vi "KB-求内环平面点.vi"(10 "offset":i32, 11 "波形图 7":dbl[](array[numeric])=[0.0, 0.0, 3.9952999999999994, 3.9923, 3.9387999999999996, 3.8314999999999997, 3.7700000000000005, 3.7629000000000006, 3.7614999999999994, 3.7604999999999995, 3.7603999999999997, 3.7639000000000005, 3.7711999999999994, 0.0]) -> (2 "index":i32, 3 "元素":dbl)   [LabVIEW 2015]
panel:
  out "x/y":dbl
  out "已排序的数组 2":dbl[](array[numeric])
  out "已排序的数组":dbl[](array[numeric])
  out "最小值 2":dbl
  out "元素索引":i32
  out "最小索引 2":i32
  out "反转的数组 3":dbl[](array[numeric])
  out "反转的数组 2":dbl[](array[numeric])
  out "反转的数组":dbl[](array[numeric])
  out "最小索引":i32
  out "波形图 6":dbl[](graph)
  out "最小值":dbl
  out "波形图 5":dbl[](graph)
  out "数组":dbl[](array[numeric])
  out "波形图 4":dynamicdata(graph)
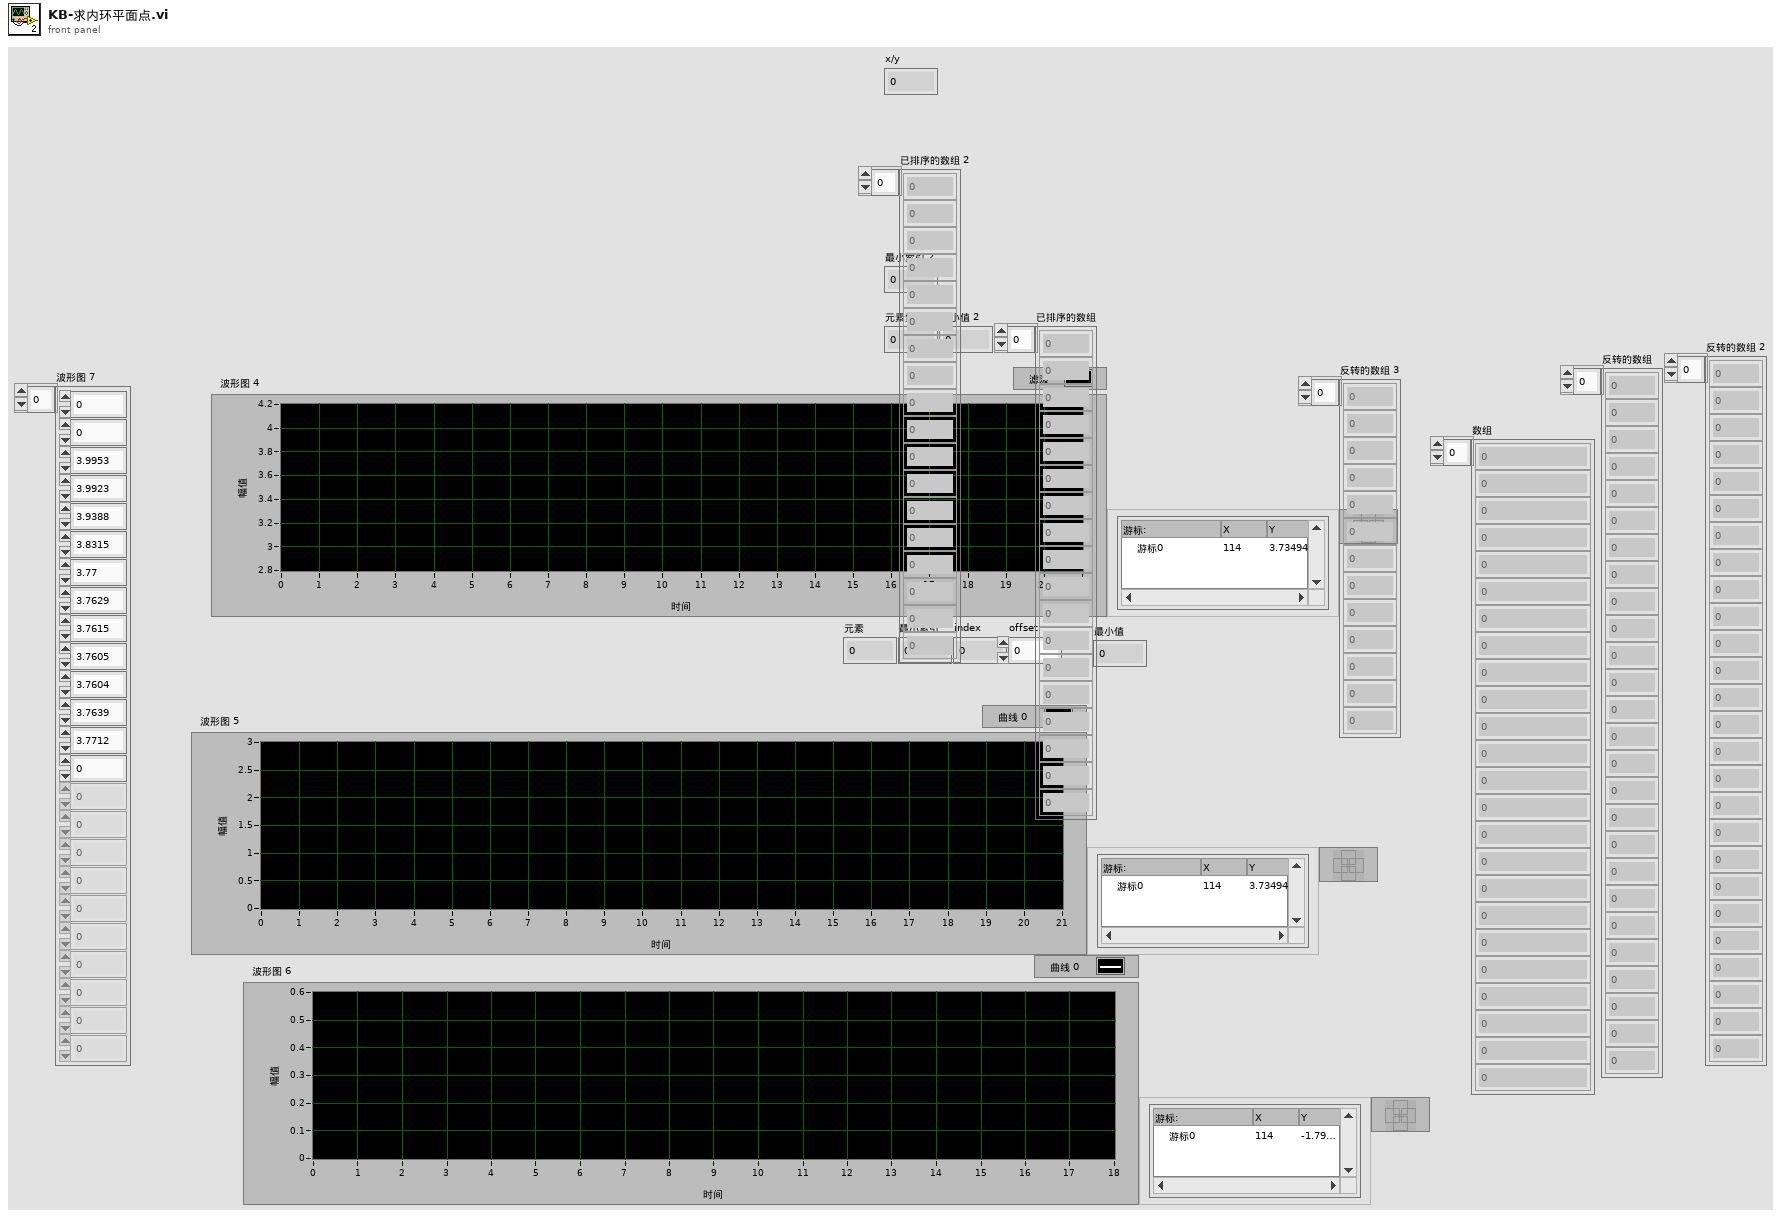
[diagram p1: front panel]
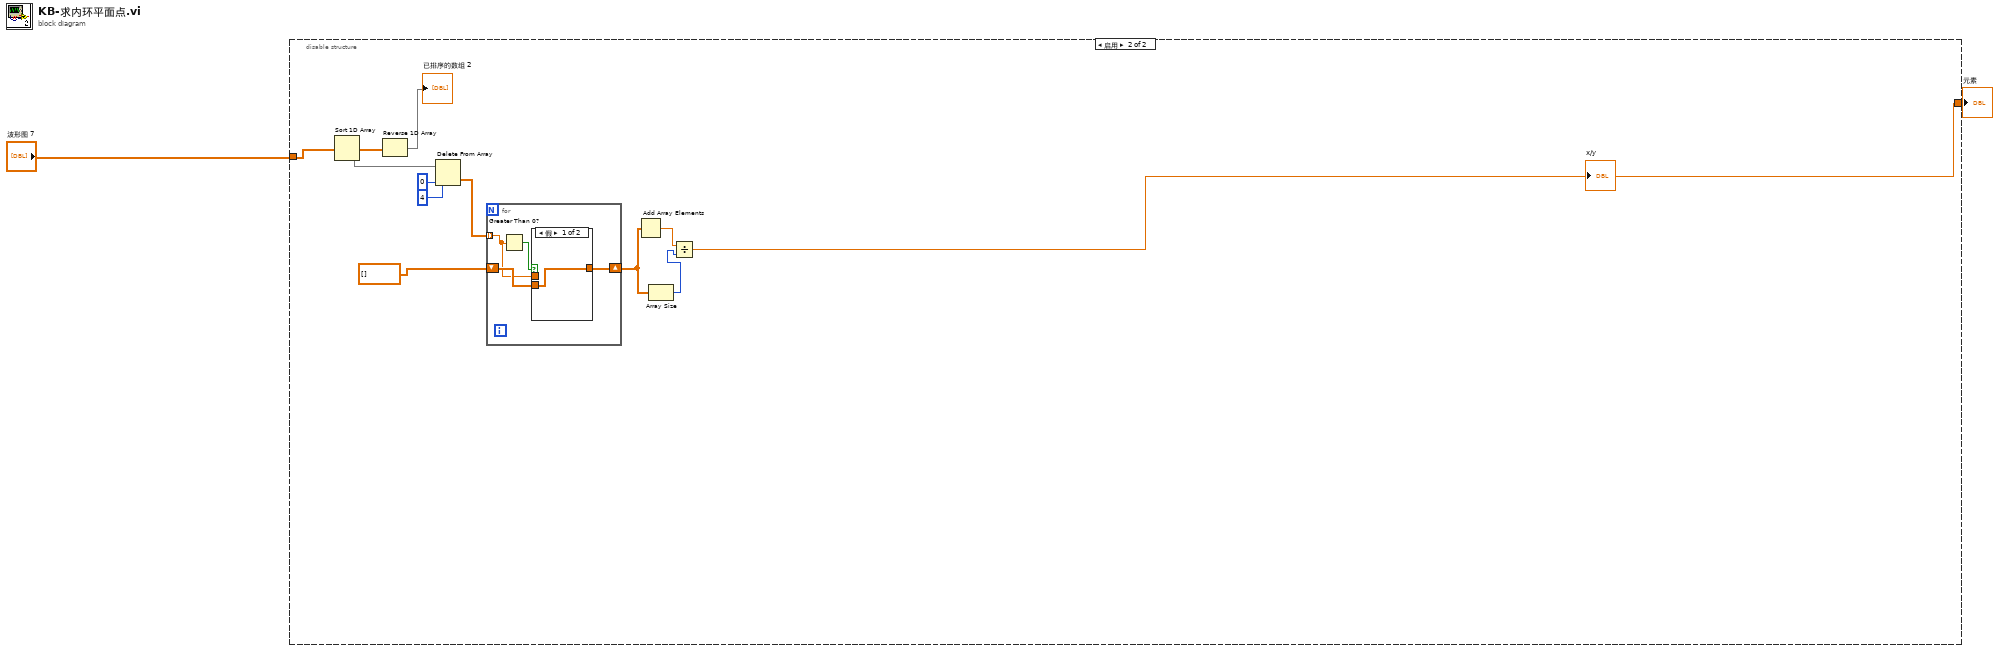
[diagram p0: block diagram]
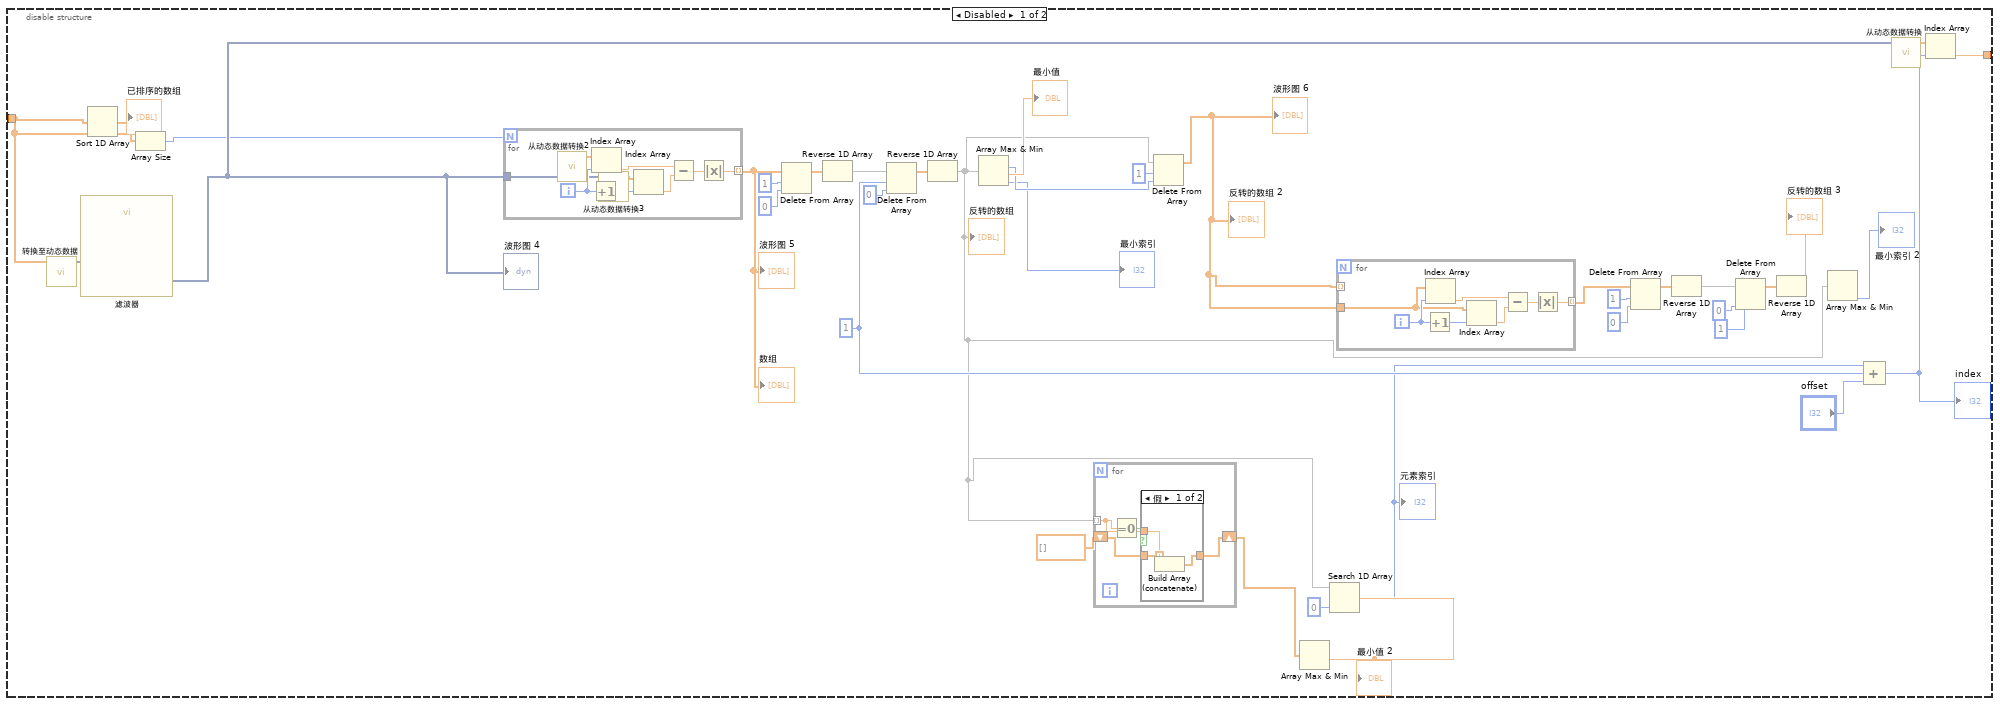
[diagram p2: hidden frame]
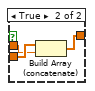
[diagram p4: hidden frame]
diagram:
  n1 = disable-structure shown="启用" {
    disable-tunnel: [w33 w69] -> w2
    disable-tunnel: "波形图 7" -> [w4 w75]
    frame Disabled {
      w32 = 1 ("长度")
      n2 = call "转换至动态数据"("Array"=w4) -> ("Dynamic Data Type"=w8:dynamicdata)  [unwired: 3 in]
      n3 = call "滤波器"("Signal"=w8) -> ("Filtered Signal"=w7:dynamicdata)  [unwired: 9 in, 1 out]
      "波形图 4" <- w7
      n4 = Sort 1D Array(array=w4) -> (sorted array=→"已排序的数组":dbl[])
      n5 = Array Size(array=w4) -> (size(s)=w5:i32)
      n6 = for {
        N: w5 -> [_]
        tunnel: w7 -> [w61]
        tunnel: [w58] -> w14 mode=indexing
        i -> [w63]
        n7 = call "从动态数据转换2"("Dynamic Data Type"=w61) -> ("Array"=w57:dbl[])  [unwired: 3 in]
        n8 = Increment(x=w63) -> (x+1=w64:i32)
        n9 = Index Array(array=w57, index=w63) -> (element=w62:dbl)
        n10 = call "从动态数据转换3"("Dynamic Data Type"=w61) -> ("Array"=w56:dbl[])  [unwired: 3 in]
        n11 = Index Array(array=w56, index=w64) -> (element=w60:dbl)
        n12 = Subtract(x=w62, y=w60) -> (x-y=w59:dbl)
        n13 = Absolute Value(x=w59) -> (abs(x)=w58:dbl)
      }
      "数组" <- w14
      "波形图 5" <- w14
      n14 = Delete From Array(array=w14, length=1 ("长度"), index=0 ("索引")) -> (array with subset deleted=w38:dbl[])  [unwired: 1 out]
      n15 = Reverse 1D Array(array=w38) -> (reversed array=w36:dbl[])
      n16 = Delete From Array(array=w36, length=w32, index=0 ("索引")) -> (array with subset deleted=w35:dbl[])  [unwired: 1 out]
      n17 = Reverse 1D Array(array=w35) -> (reversed array=w10:dbl[])
      "反转的数组" <- w10
      n18 = Array Max & Min(array=w10) -> (max index (indices)=w29:i32, min value=→"最小值":dbl, min index (indices)=→"最小索引":i32)  [unwired: 1 out]
      n19 = for {
        shift-right: [w42] -> w11
        shift-left: dbl[] [] -> [w43]
        tunnel: w10 -> [w41] mode=indexing
        n20 = Equal To 0?(x=w41) -> (x = 0?=w44:bool)
        n21 = case shown="假" w44 {
          tunnel: w43 -> [w47 w48]
          tunnel: [w46 w48] -> w42
          tunnel: w41 -> [w45 _]
          frame False {
            n22 = Build Array (concatenate)(w47, w45) -> (w46:dbl[])
          }
          frame True {
          }
        }
      }
      n23 = Delete From Array(array=w10, length=1 ("长度"), index=w29) -> (array with subset deleted=w27:dbl[])  [unwired: 1 out]
      "波形图 6" <- w27
      "反转的数组 2" <- w27
      n24 = Array Max & Min(array=w11) -> (min value=w13:dbl)  [unwired: 3 out]
      "最小值 2" <- w13
      n25 = Search 1D Array(1D array=w10, element=w13, start index (0)=0 ("开始索引(0)")) -> (index of element=w9:i32)
      "元素索引" <- w9
      n26 = for {
        tunnel: w27 -> [w52]
        tunnel: [w49] -> w20 mode=indexing
        tunnel: w27 -> [_] mode=indexing
        i -> [w54]
        n27 = Increment(x=w54) -> (x+1=w55:i32)
        n28 = Index Array(array=w52, index=w54) -> (element=w53:dbl)
        n29 = Index Array(array=w52, index=w55) -> (element=w51:dbl)
        n30 = Subtract(x=w53, y=w51) -> (x-y=w50:dbl)
        n31 = Absolute Value(x=w50) -> (abs(x)=w49:dbl)
      }
      n32 = Delete From Array(array=w20, length=1 ("长度"), index=0 ("索引")) -> (array with subset deleted=w22:dbl[])  [unwired: 1 out]
      n33 = Reverse 1D Array(array=w22) -> (reversed array=w24:dbl[])
      n34 = Delete From Array(array=w24, length=1 ("长度"), index=0 ("索引")) -> (array with subset deleted=w25:dbl[])  [unwired: 1 out]
      n35 = Reverse 1D Array(array=w25) -> (reversed array=→"反转的数组 3":dbl[])
      n36 = Array Max & Min(array=w10) -> (min index (indices)=→"最小索引 2":i32)  [unwired: 3 out]
      n37 = Compound Arithmetic op=ADD(w9, w32, "offset") -> (w31:i32)
      "index" <- w31
      n38 = call "从动态数据转换"("Dynamic Data Type"=w7) -> ("Array"=w6:dbl[])  [unwired: 3 in]
      n39 = Index Array(array=w6, index=w31) -> (element=w33:dbl)
    }
    frame Enabled {
      n40 = Sort 1D Array(array=w75) -> (sorted array=w74:dbl[])
      n41 = Reverse 1D Array(array=w74) -> (reversed array=w73:dbl[])
      "已排序的数组 2" <- w73
      n42 = Delete From Array(array=w73, length=4 ("长度"), index=0 ("索引")) -> (deleted portion=w68:dbl[])  [unwired: 1 out]
      n43 = for {
        tunnel: w68 -> [w77] mode=indexing
        shift-right: [w76] -> w66
        shift-left: dbl[] [] -> [w78]
        n44 = Greater Than 0?(x=w77) -> (x > 0?=w79:bool)
        n45 = case shown="假" w79 {
          tunnel: w78 -> [w80 w83]
          tunnel: w77 -> [_ w82]
          tunnel: [w80 w81] -> w76
          frame False {
          }
          frame True {
            n46 = Build Array (concatenate)(w83, w82) -> (w81:dbl[])
          }
        }
      }
      n47 = Add Array Elements(numeric array=w66) -> (sum=w71:dbl)
      n48 = Array Size(array=w66) -> (size(s)=w65:i32)
      n49 = Divide(x=w71, y=w65) -> (x/y=w69:dbl)
      "x/y" <- w69
    }
  }
  "元素" <- w2
